vi "FMA1600A Send Receive.vi"(7 "Unit ID":string, 8 "error in (no error)":errorcluster, 9 "Gas Type":T1, 10 "FMA1600A Commands":T2, 11 "VISA Refnum in":refnum<visa-resource-name>) -> (0 "error out":errorcluster, 2 "Raw FMA1600A Data":string, 3 "VISA Refnum out":refnum<visa-resource-name>)   [LabVIEW 2023]
uses:
  Type Definitions/FMA1600A Commands.ctl
  Type Definitions/FMA1600A Gas Type.ctl
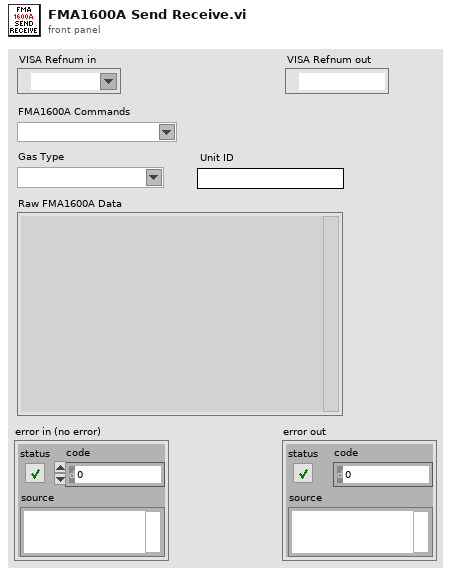
[diagram p1: front panel]
types:
  T1 = typedef "FMA1600A Gas Type.ctl" = string
  T2 = typedef "FMA1600A Commands.ctl" = string
  T3 = typedef "FMA1600A Data.ctl" = cluster{"Pressure (PSIA)":dbl, "Temperature (°F)":dbl, "Vol. Flow (LPM)":dbl, "Mass Flow (SLPM)":dbl, "Gas Type":string, "Tot. Flow (Liters)":dbl, "Meter ID":string}
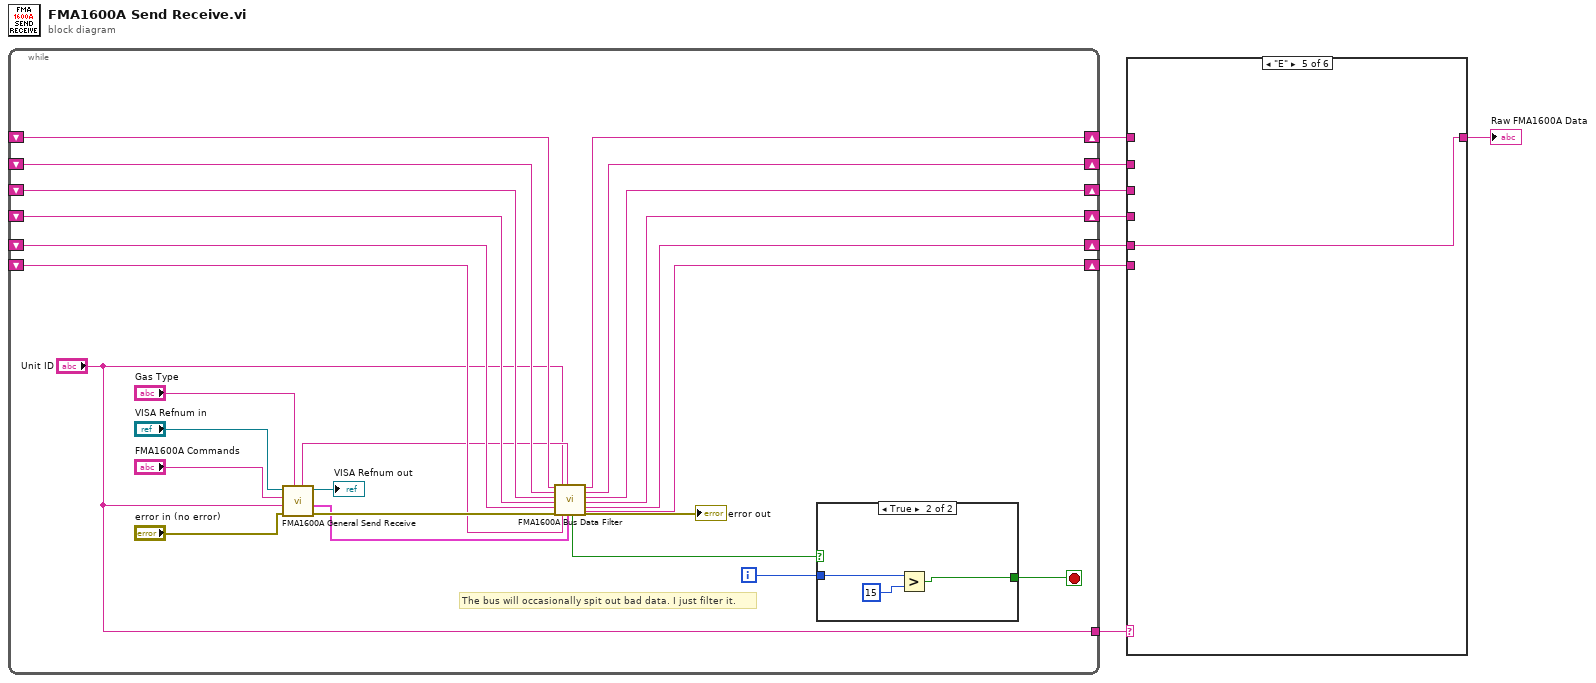
[diagram p0: block diagram]
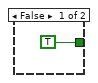
[diagram p7: hidden frame]
diagram:
  n1 = while {
    shift-right: [w25] -> w8
    shift-left: _ -> [w26]
    shift-right: [w23] -> w6
    shift-left: _ -> [w24]
    shift-right: [w22] -> w5
    shift-left: _ -> [w21]
    shift-right: [w19] -> w4
    shift-left: _ -> [w20]
    shift-right: [w17] -> w3
    shift-left: _ -> [w18]
    shift-right: [w15] -> w2
    shift-left: _ -> [w16]
    tunnel: ["Unit ID"] -> w1
    i -> [w31]
    stop <- w30 stop-if-true
    # "The bus will occasionally spit out bad data. I just filter it."
    n2 = call "FMA1600A General Send Receive.vi"("Gas Type"="Gas Type", "error in (no error)"="error in (no error)", "Unit ID in"="Unit ID", "FMA1600A Commands"="FMA1600A Commands", "VISA Refnum in"="VISA Refnum in") -> ("error out"=w28:errorcluster, "FMA1600A Gas Data"=w14:T3, "VISA Refnum out"=→"VISA Refnum out":refnum<visa-resource-name>, "Data Stream"=w13:string)  [unwired: 3 in]
    n3 = call "FMA1600A Bus Data Filter.vi"("Station A Input"=w26, "Station B Input"=w24, "Station C Input"=w21, "Station D Input"=w20, "Station E Input"=w18, "Error In"=w28, "Unit ID"="Unit ID", "Station F Input"=w16, "Data Stream"=w13, "FMA1600A Gas Data"=w14) -> ("Check Shutdown"=w12:bool, "Station F Output"=w15:string, "Station A Output"=w25:string, "Station B Output"=w23:string, "Station C Output"=w22:string, "Station D Output"=w19:string, "Station E Output"=w17:string, "Error Out"=→"error out":errorcluster)  [unwired: 2 in]
    n4 = case shown="True" w12 {
      tunnel: [TRUE ("y") w35] -> w30
      tunnel: w31 -> [_ w36]
      frame False {
      }
      frame True {
        n5 = Greater?(x=w36, y=15) -> (0:w35:bool)
      }
    }
  }
  n6 = case shown="\"E\"" w1 {
    tunnel: [w38 w39 w40 w41 w42 w43] -> w7
    tunnel: w8 -> [w38 _ _ _ _ _]
    tunnel: w6 -> [_ w39 _ _ _ _]
    tunnel: w5 -> [_ _ w40 _ _ _]
    tunnel: w4 -> [_ _ _ w41 _ _]
    tunnel: w3 -> [_ _ _ _ w42 _]
    tunnel: w2 -> [_ _ _ _ _ w43]
    frame "A", Default {
    }
    frame "B" {
    }
    frame "C" {
    }
    frame "D" {
    }
    frame "E" {
    }
    frame "F" {
    }
  }
  "Raw FMA1600A Data" <- w7
